vi "打开通讯连接.vi"(11 "界面控件引用":T1) -> (3 "连接成功":bool)   [LabVIEW 2017]
panel:
  out "error out":errorcluster
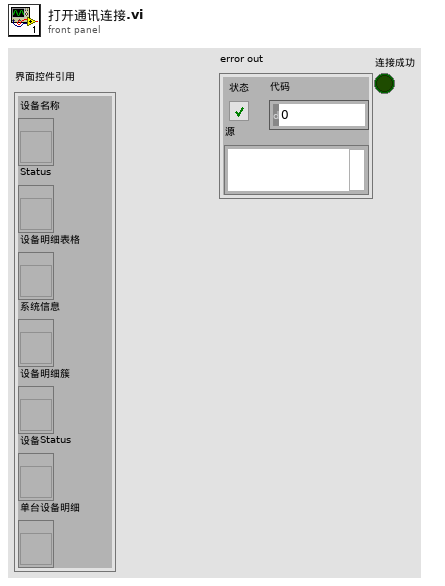
[diagram p1: front panel]
types:
  T1 = typedef "界面控件引用.ctl" = cluster{"设备名称":refnum<vi>, "Status":refnum<vi>, "设备明细表格":refnum<vi>, "系统信息":refnum<vi>, "设备明细簇":refnum<vi>, "设备Status":refnum<vi>, "单台设备明细":refnum<vi>}
  T2 = typedef "单台设备明细.ctl" = cluster{"设备名称":string, "IP地址":string, "允许开机":bool, "允许连接":bool, "允许归零":bool, "允许自动":bool, "允许退出":bool, "允许关机":bool, "connection ID":refnum<k5>}
  T3 = typedef "Status.ctl" = cluster{"开机":bool, "连接":bool, "归零":bool, "自动":bool, "退出":bool, "关机":bool}
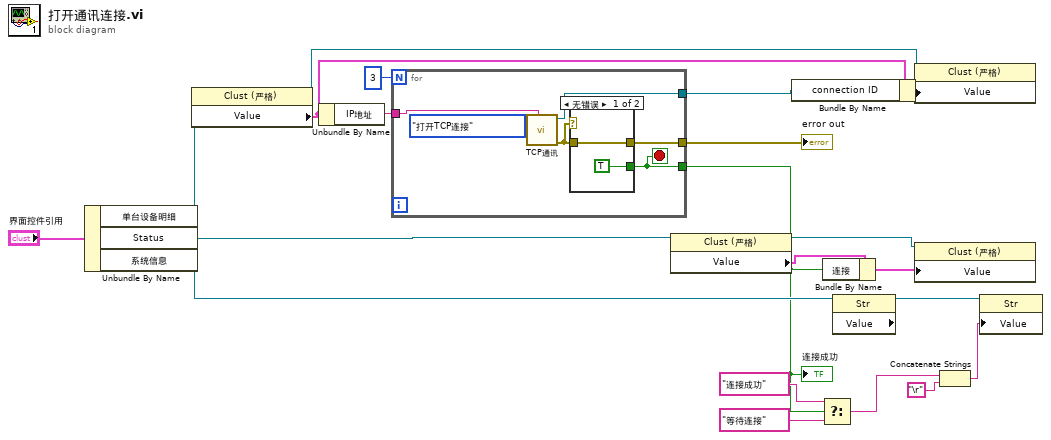
[diagram p0: block diagram]
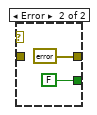
[diagram p2: hidden frame]
diagram:
  n1 = Unbundle By Name("界面控件引用") -> ("单台设备明细"=w18:refnum<vi>, "Status"=w6:refnum<vi>, "系统信息"=w12:refnum<vi>)
  n2 = property class="Clust (严格)"(reference=w18) -> (reference out=w20:refnum<vi>, "Value"=w8:T2)  [unwired: 1 in, 1 out]
  n3 = Unbundle By Name(w8) -> ("IP地址"=w19:string)
  n4 = for {
    N: 3 -> [_]
    tunnel: [w27] -> w21
    tunnel: w19 -> [w26]
    tunnel: [w25] -> w16
    tunnel: [w23] -> w3
    stop <- w23 stop-if-true
    n5 = call "TCP通讯.vi"("service name"=w26, "选项"=enum16{"NA", "侦听", "读取", "写入", "关闭", "打开TCP连接"}."打开TCP连接") -> ("error out"=w24:errorcluster, "connection ID out"=w27:refnum<k5>)  [unwired: 5 in, 3 out]
    n6 = case shown="无错误" w24 {
      tunnel: [TRUE FALSE] -> w23
      tunnel: [w28 errorcluster {"status"=FALSE, "code"=0, "source"=""} ("error out")] -> w25
      tunnel: w24 -> [w28 _]
      frame No Error {
      }
      frame Error {
      }
    }
  }
  "error out" <- w16
  "连接成功" <- w3
  n7 = property class="Clust (严格)"(reference=w6) -> (reference out=w2:refnum<vi>, "Value"=w5:T3)  [unwired: 1 in, 1 out]
  n8 = Bundle By Name(cluster=w8, "connection ID"=w21) -> (w7:T2)
  n9 = Select(t="连接成功", s=w3, f="等待连接") -> (s? t:f=w11:string)
  n10 = Bundle By Name(cluster=w5, "连接"=w3) -> (w4:T3)
  n11 = property class="Str" props=["Value"](reference=w12) -> (reference out=w1:refnum<vi>)  [unwired: 1 in, 2 out]
  n12 = property class="Clust (严格)"(reference=w20, "Value"=w7) -> ()  [unwired: 1 in, 2 out]
  n13 = property class="Clust (严格)"(reference=w2, "Value"=w4) -> ()  [unwired: 1 in, 2 out]
  n14 = Concatenate Strings(w11, "\r") -> (w10:string)
  n15 = property class="Str"(reference=w1, "Value"=w10) -> ()  [unwired: 1 in, 2 out]
